vi "Test Array VIs.vi"() -> ()   [LabVIEW 2014]
uses:
  <vilib>/measure/NI_MABase.lvlib
panel:
  out "Waveform Graph 2":dbl[](graph)
  out "Waveform Graph":waveform(dbl)(graph)
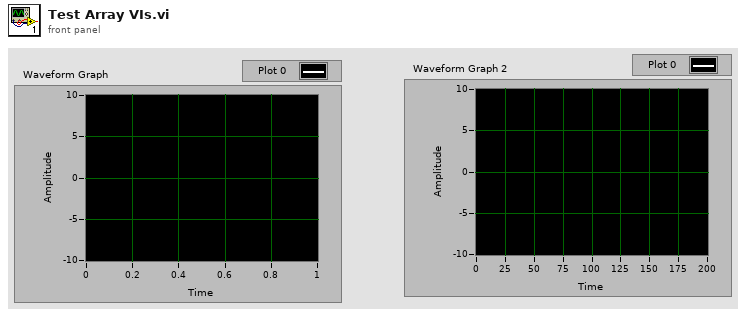
[diagram p1: front panel]
types:
  T1 = enum16{"Sine Wave", "Triangle Wave", "Square Wave", "Sawtooth Wave"}
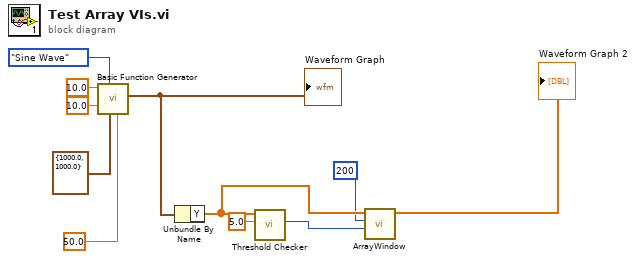
[diagram p0: block diagram]
diagram:
  n1 = call <vilib>:"Basic Function Generator.vi"("square wave duty cycle (%)"=50.0, "sampling info"=cluster{"Fs":dbl, "#s":dbl} {"Fs"=1000.0, "#s"=1000.0}, "signal type"=T1."Sine Wave", "amplitude"=10.0, "frequency"=10.0) -> ("signal out"=w6:waveform(dbl))  [unwired: 4 in, 2 out]
  "Waveform Graph" <- w6
  n2 = Unbundle By Name(w6) -> ("Y"=w3:dbl[])
  n3 = call "Threshold Checker.vi"("Threshold"=5.0, "Data"=w3) -> ("Index of Value = to or exceeding threshold"=w4:i32)  [unwired: 7 in, 2 out]
  n4 = call "ArrayWindow.VI"("Index"=w4, "Total amount of Pts"=200, "Input Y-values"=w3) -> ("Output Array"=→"Waveform Graph 2":dbl[])  [unwired: 8 in]
